vi "FGV_Initialization.vi"(8 "error in (no error)":errorcluster) -> (0 "error out":errorcluster)   [LabVIEW 2025]
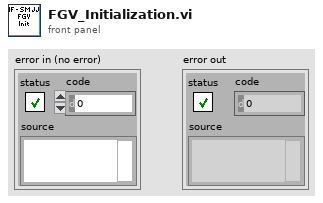
[diagram p1: front panel]
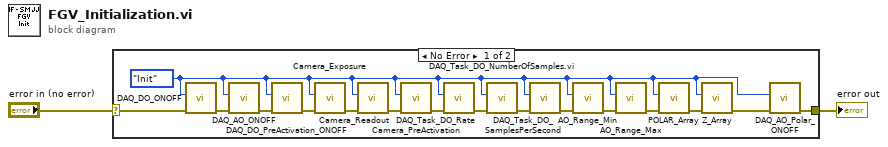
[diagram p0: block diagram]
diagram:
  n1 = case shown="No Error" "error in (no error)" {
    selector: "error in (no error)" -> [w4 w19]
    tunnel: [w9 w19] -> w2
    frame No Error {
      w3 = enum16{"Init", "Write", "Read"}."Init" ("Action")
      n2 = call "DAQ_DO_ONOFF.vi"("error in"=w4, "Action"=w3) -> ("error out"=w12:errorcluster)  [unwired: 8 in, 1 out]
      n3 = call "DAQ_AO_ONOFF.vi"("error in"=w12, "Action"=w3) -> ("error out"=w11:errorcluster)  [unwired: 8 in, 1 out]
      n4 = call "DAQ_DO_PreActivation_ONOFF.vi"("error in"=w11, "Action"=w3) -> ("error out"=w18:errorcluster)  [unwired: 8 in, 1 out]
      n5 = call "Camera_Exposure.vi"("error in"=w18, "Action"=w3) -> ("error out"=w16:errorcluster)  [unwired: 8 in, 1 out]
      n6 = call "Camera_Readout.vi"("error in"=w16, "Action"=w3) -> ("error out"=w17:errorcluster)  [unwired: 8 in, 1 out]
      n7 = call "Camera_PreActivation.vi"("error in"=w17, "Action"=w3) -> ("error out"=w14:errorcluster)  [unwired: 8 in, 1 out]
      n8 = call "DAQ_Task_DO_Rate.vi"("error in"=w14, "Action"=w3) -> ("error out"=w15:errorcluster)  [unwired: 8 in, 1 out]
      n9 = call "DAQ_Task_DO_NumberOfSamples.vi.vi"("error in"=w15, "Action"=w3) -> ("error out"=w13:errorcluster)  [unwired: 8 in, 1 out]
      n10 = call "DAQ_Task_DO_SamplesPerSecond.vi"("error in"=w13, "Action"=w3) -> ("error out"=w5:errorcluster)  [unwired: 8 in, 1 out]
      n11 = call "AO_Range_Min.vi"("error in"=w5, "Action"=w3) -> ("error out"=w6:errorcluster)  [unwired: 8 in, 1 out]
      n12 = call "AO_Range_Max.vi"("error in"=w6, "Action"=w3) -> ("error out"=w10:errorcluster)  [unwired: 8 in, 1 out]
      n13 = call "POLAR_Array.vi"("error in"=w10, "Action"=w3) -> ("error out"=w8:errorcluster)  [unwired: 8 in, 1 out]
      n14 = call "Z_Array.vi"("error in"=w8, "Action"=w3) -> ("error out"=w7:errorcluster)  [unwired: 8 in, 1 out]
      n15 = call "DAQ_AO_Polar_ONOFF.vi"("error in"=w7, "Action"=w3) -> ("error out"=w9:errorcluster)  [unwired: 8 in, 1 out]
    }
    frame Error {
    }
  }
  "error out" <- w2
